vi "PriceData to Waveform.vi"(10 "PriceData_RealTime":T1, 11 "Max Forecast Length":i32) -> (3 "Waveform":waveform(dbl))   [LabVIEW 2018, in "Generic Optimization Actor.lvlib" / "Generic Optimization.lvclass"]
uses:
  Generic Optimization.lvclass
  <vilib>/ORNL/CSEISMIC DDS/CSEISMIC DDS Base/Data Types/PriceData_RealTime.ctl
  <vilib>/ORNL/CSEISMIC DDS/CSEISMIC DDS Base/Data Types/Controls/DeviceID.ctl
  <vilib>/ORNL/CSEISMIC DDS/CSEISMIC DDS Base/CSEISMIC DDS.lvclass
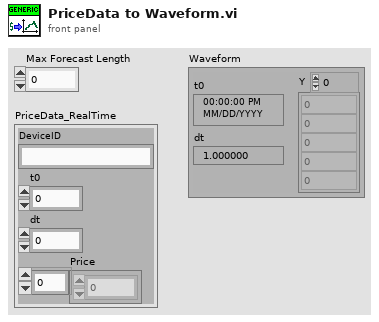
[diagram p1: front panel]
types:
  T1 = typedef "CSEISMIC DDS.lvlib/CSEISMIC DDS.lvclass/PriceData_RealTime.ctl" = cluster{"DeviceID":T2, "t0":dbl, "dt":dbl, "Price":dbl[]}
  T2 = typedef "CSEISMIC DDS.lvlib/CSEISMIC DDS.lvclass/DeviceID.ctl" = string
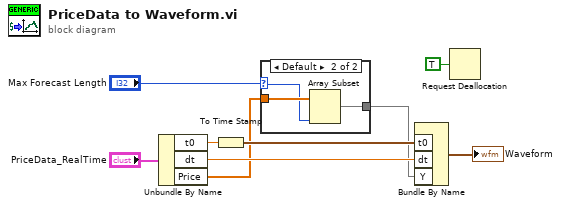
[diagram p0: block diagram]
diagram:
  n1 = Unbundle By Name("PriceData_RealTime") -> ("t0"=w7:dbl, "dt"=w8:dbl, "Price"=w4:dbl[])
  n2 = To Time Stamp(1:w7) -> (0:w6:timestamp)
  n3 = case shown="Default" "Max Forecast Length" {
    selector: "Max Forecast Length" -> [_ w11]
    tunnel: w4 -> [w10 w13]
    tunnel: [w10 w12] -> w3
    frame -1 {
    }
    frame Default {
      n4 = Array Subset(array=w13, length=w11) -> (w12:dbl[])  [unwired: 1 in]
    }
  }
  n5 = Bundle By Name("t0"=w6, "dt"=w8, "Y"=w3) -> (→"Waveform":waveform(dbl))  [unwired: 1 in]
  n6 = Request Deallocation(TRUE ("flag")) -> ()
